vi "Get Start Point.vi"(8 "error in (no error)":errorcluster, 11 "Graphics Object.lvclass in":refnum<class "Graphics Object.lvclass">) -> (0 "error out":errorcluster, 2 "start point":cluster{"x":i16, "y":i16}, 3 "Graphics Object.lvclass out":refnum<class "Graphics Object.lvclass">)   [LabVIEW 2020, in "Graphics Object.lvclass"]
doc: "Get the start point of a bounding box surrounding a graphics object"
uses:
  Graphics Object.lvclass
  Graphics Object.lvclass/Graphics Object.ctl
panel:
  # "expressionflow.com"
  # "Copyright (c) 2008 Tomi Maila. All rights reserved."
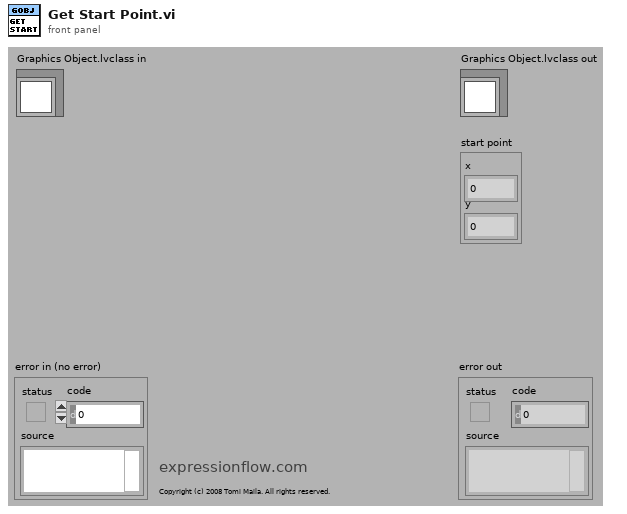
[diagram p1: front panel]
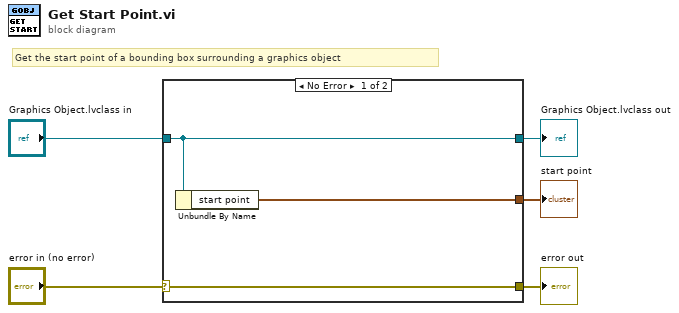
[diagram p0: block diagram]
diagram:
  # "Get the start point of a bounding box surrounding a graphics object"
  n1 = case shown="No Error" "error in (no error)" {
    selector: "error in (no error)" -> [w8 w9]
    tunnel: [w8 w9] -> w4
    tunnel: [w7 w10] -> w2
    tunnel: "Graphics Object.lvclass in" -> [w7 w10]
    tunnel: [w6 _] -> w1
    frame No Error {
      n2 = Unbundle By Name(w7) -> ("start point"=w6:cluster{"x":i16, "y":i16})
    }
    frame Error {
    }
  }
  "error out" <- w4
  "Graphics Object.lvclass out" <- w2
  "start point" <- w1
